vi "ComputerName.vi"() -> (2 "ComputerName":string)   [LabVIEW 2020]
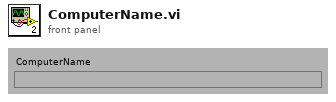
[diagram p1: front panel]
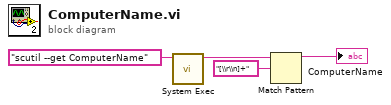
[diagram p0: block diagram]
diagram:
  n1 = call <vilib>:"System Exec.vi"("command line"="scutil --get ComputerName") -> ("standard output"=w3:string)  [unwired: 7 in, 3 out]
  n2 = Match Pattern(string=w3, regular expression="[\\r\\n]+") -> (before substring=→"ComputerName":string)  [unwired: 1 in, 3 out]
